vi "hamamatsuReadToRAM.vi"(0 "waitOnStartAcquisition":bool) -> (1 "frames":u16[][][](array[numeric]), 2 "frameCount":i32[](array[numeric]), 3 "frameSum":dbl[](array[numeric]))   [LabVIEW 2017]
doc: "Reads frames from the Hamamatsu camera to RAM. If hamamatsuStartTriggerMode is set to true, the camera waits for a hardware trigger to start. If waitOnStartAcquisition is set to true, the camera waits for a software start (acquisitionStart set to true). Otherwise, it starts the acquisition immediately.\n\nThe acquisition loop stops with an acquisitionStop (or a generalStop)."
uses:
  globalUtilities.vi
  globalDevices.vi
  <vilib>/Analysis/NI_AALBase.lvlib
panel:
  # "Remember to inline the subVI into the caller when using this\nVI, otherwise the output frames will have to be copied to be\nreturned to the caller."
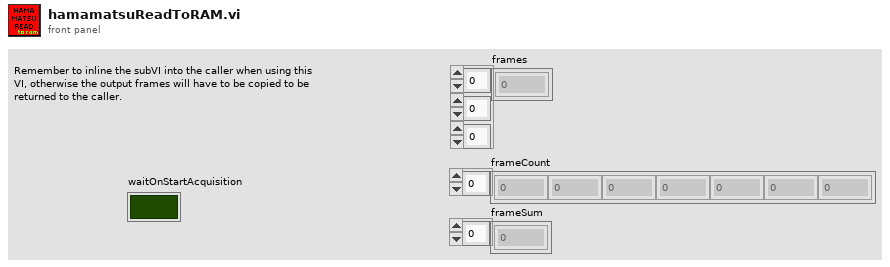
[diagram p1: front panel]
types:
  T1 = enum16{"big-endian, network order", "native, host order", "little-endian"}
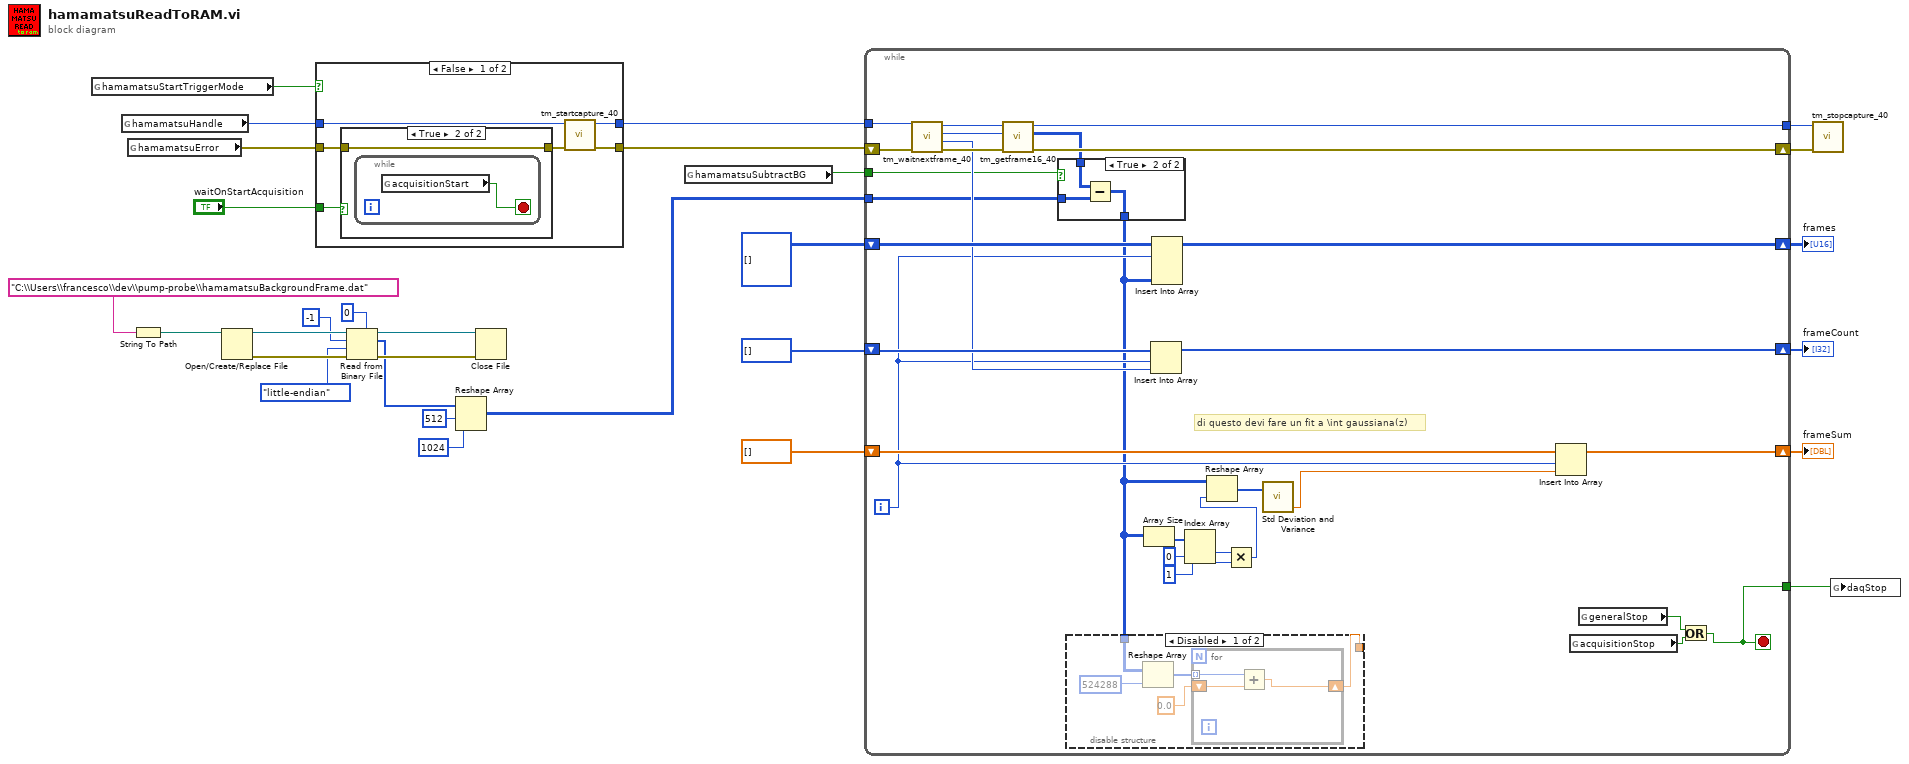
[diagram p0: block diagram]
diagram:
  n1 = global read "globalDevices.vi" "hamamatsuStartTriggerMode"() -> (w29:bool)
  n2 = global read "globalDevices.vi" "hamamatsuHandle"() -> (w28:u32)
  n3 = global read "globalDevices.vi" "hamamatsuError"() -> (w27:errorcluster)
  n4 = String To Path(string="C:\\Users\\francesco\\dev\\pump-probe\\hamamatsuBackgroundFrame.dat") -> (path=w12:path)
  n5 = Open/Create/Replace File(file path (use dialog)=w12) -> (refnum out=w11:refnum<file>, error out=w10:errorcluster)  [unwired: 5 in, 1 out]
  n6 = case shown="False" w29 {
    tunnel: w28 -> [w35 w40]
    tunnel: w27 -> [w31 w39]
    tunnel: [w34 w40] -> w26
    tunnel: [w33 w39] -> w25
    tunnel: "waitOnStartAcquisition" -> [w32 _]
    frame False {
      n7 = case shown="True" w32 {
        tunnel: w31 -> [w36 w37]
        tunnel: [w36 w37] -> w30
        frame False {
        }
        frame True {
          n8 = while {
            stop <- w38 stop-if-true
            n9 = global read "globalUtilities.vi" "acquisitionStart"() -> (w38:bool)
          }
        }
      }
      n10 = call <userlib>:"tm_startcapture_40.vi"("error in (no error)"=w30, "Handle in"=w35) -> ("error out"=w33:errorcluster, "Handle out"=w34:u32)  [unwired: 8 in]
    }
    frame True {
    }
  }
  n11 = Read from Binary File(5:u16 0, 8:w10, 9:T1."little-endian" ("byte order (0:big-endian, network order)"), 10:-1 ("count (1)"), 11:w11) -> (0:w5:errorcluster, 2:w4:u16[], 3:w6:refnum<file>)  [unwired: 1 in, 1 out]
  n12 = Reshape Array(w4, 512 ("dimension size"), 1024 ("dimension size")) -> (w1:u16[][])
  n13 = Close File(refnum=w6, error in=w5) -> ()  [unwired: 2 out]
  n14 = global read "globalDevices.vi" "hamamatsuSubtractBG"() -> (w14:bool)
  n15 = while {
    tunnel: w26 -> [w70]
    tunnel: [w65] -> w17
    shift-right: [w64] -> w18
    shift-left: w25 -> [w69]
    shift-right: [w60] -> w21
    shift-left: u16[][][] [] -> [w63]
    shift-right: [w59] -> w20
    shift-left: i32[] [] -> [w62]
    tunnel: [w53] -> w15
    shift-right: [w56] -> w19
    shift-left: dbl[] [] -> [w58]
    tunnel: w14 -> [w44]
    tunnel: w1 -> [w42]
    i -> [w57]
    stop <- w53 stop-if-true
    # "di questo devi fare un fit a \\int gaussiana(z)"
    n16 = call <userlib>:"tm_waitnextframe_40.vi"("error in (no error)"=w69, "Handle in"=w70) -> ("error out"=w67:errorcluster, "Frame Count"=w61:i32, "Frame Index"=w66:i32, "Handle out"=w68:u32)  [unwired: 6 in]
    n17 = call <userlib>:"tm_getframe16_40.vi"("error in (no error)"=w67, "Frame Index"=w66, "Handle in"=w68) -> ("error out"=w64:errorcluster, "Data"=w43:u16[][], "Handle out"=w65:u32)  [unwired: 5 in, 1 out]
    n18 = case shown="True" w44 {
      tunnel: w43 -> [w71 w74]
      tunnel: w42 -> [_ w73]
      tunnel: [w71 w72] -> w41
      frame False {
      }
      frame True {
        n19 = Subtract(x=w74, y=w73) -> (x-y=w72:u16[][])
      }
    }
    n20 = disable-structure shown="Disabled" {
      disable-tunnel: w41 -> [w79 _]
      disable-tunnel: [w75 _] -> _
      frame Disabled {
        n21 = Reshape Array(w79, 524288) -> (w77:u16[])
        n22 = for {
          tunnel: w77 -> [w82] mode=indexing
          shift-right: [w80] -> w75
          shift-left: 0.0 -> [w81]
          n23 = Add(x=w82, y=w81) -> (x+y=w80:dbl)
        }
      }
      frame Enabled {
      }
    }
    n24 = Array Size(array=w41) -> (size(s)=w51:i32[])
    n25 = Insert Into Array(array=w62, index=w57, new element=w61) -> (w59:i32[])
    n26 = Insert Into Array(array=w63, index (dim 0)=w57, new element=w41) -> (w60:u16[][][])  [unwired: 2 in]
    n27 = Index Array(array=w51, index #1=0 ("index"), index #2=1 ("index")) -> (element #1=w48:i32, element #2=w47:i32)
    n28 = Multiply(x=w48, y=w47) -> (x*y=w46:i32)
    n29 = Reshape Array(w41, w46) -> (w52:u16[])
    n30 = call <vilib>:"Std Deviation and Variance.vi"("X"=w52) -> ("variance"=w45:dbl)  [unwired: 1 in, 2 out]
    n31 = Insert Into Array(array=w58, index=w57, new element=w45) -> (w56:dbl[])
    n32 = global read "globalUtilities.vi" "acquisitionStop"() -> (w55:bool)
    n33 = global read "globalUtilities.vi" "generalStop"() -> (w54:bool)
    n34 = Or(x=w54, y=w55) -> (x .or. y?=w53:bool)
  }
  "frames" <- w21
  "frameCount" <- w20
  "frameSum" <- w19
  n35 = call <userlib>:"tm_stopcapture_40.vi"("error in (no error)"=w18, "Handle in"=w17) -> ()  [unwired: 8 in, 2 out]
  n36 = global write "globalUtilities.vi" "daqStop"(w15) -> ()
